vi "Receive Messages from Queue.vi"() -> ()   [LabVIEW 2015]
doc: "Demonstrates how to receive messages from an existing Amazon SQS queue."
uses:
  Core/HTTP Request/Region.ctl
  Core/HTTP Request/AWS Credentials.ctl
  Queue/Message.ctl
  Queue/Message Attribute Value Pair.ctl
  Queue/Message Attribute.ctl
  Queue/Custom Attribute.ctl
  Queue/Custom Attribute Type.ctl
  Queue/Queue Attribute.ctl
  Queue/Queue.lvclass
  Core/HTTP Request/HTTP Request.lvclass
panel:
  out "Messages":i32(listbox)
  in  "Region":T1
  in  "Secret Key":string
  in  "Access Key":string
  in  "Queue Name":string
  # "Overview: Demonstrates how to receive messages from an existing Amazon SQS queue.\nRequirements: LabVIEW AWS Toolkit and a registered Amazon AWS account\nInstructions:\n1. Specify the Access Key and Secret Key for your AWS account. You can create an account at http://aws.amazon.com.\n2. Specify a Region and Queue Name for the queue from which you want to receive messages.\n3. Run the VI. All the messages associated with your queue should be listed in the Messages indicator."
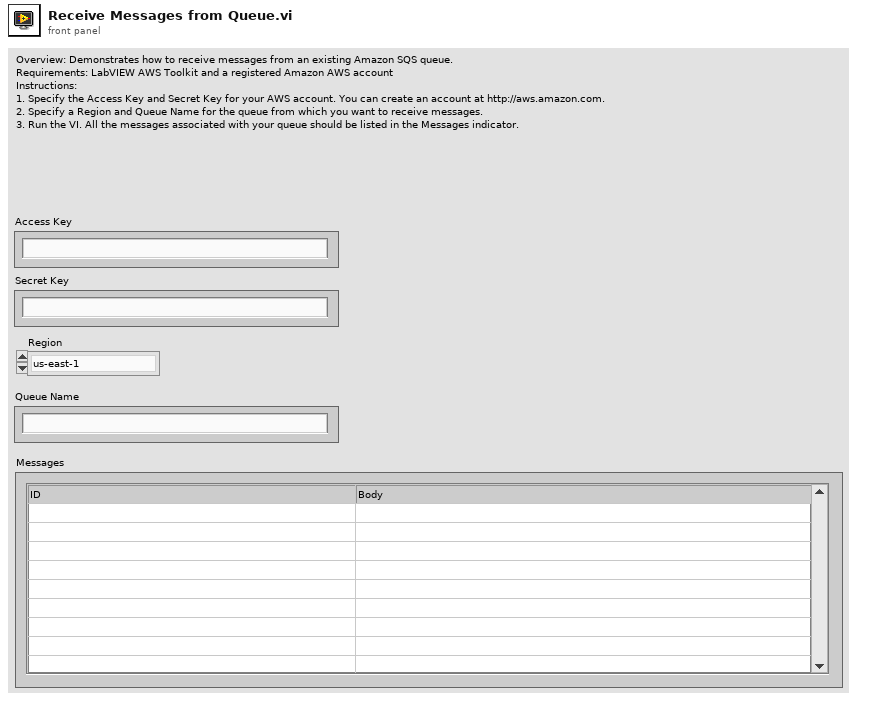
[diagram p1: front panel]
types:
  T1 = typedef "NI_AWS_Core.lvlib/HTTP Request.lvclass/Region.ctl" = enum16{"us-east-1", "us-east-2", "us-west-1", "us-west-2", "ap-northeast-1", "ap-northeast-2", "ap-southeast-1", "ap-southeast-2", "ca-central-1", "eu-central-1", "eu-west-1", "eu-west-2", "sa-east-1"}
  T2 = typedef "NI_AWS_SQS.lvlib/Queue.lvclass/Message.ctl" = cluster{"Body":string, "MD5 of Body":string, "ID":string, "Receipt Handle":string, "Native Attributes":T3[], "Custom Attributes":T5[], "MD5 of Custom Attributes":string}
  T3 = typedef "NI_AWS_SQS.lvlib/Queue.lvclass/Message Attribute Value Pair.ctl" = cluster{"Attribute":T4, "Value":string}
  T4 = typedef "NI_AWS_SQS.lvlib/Queue.lvclass/Message Attribute.ctl" = enum16{"SenderId", "SentTimestamp", "ApproximateReceiveCount", "ApproximateFirstReceiveTimestamp"}
  T5 = typedef "NI_AWS_SQS.lvlib/Queue.lvclass/Custom Attribute.ctl" = cluster{"Name":string, "Type":T6, "Value":string}
  T6 = typedef "NI_AWS_SQS.lvlib/Queue.lvclass/Custom Attribute Type.ctl" = enum16{"String", "Number", "Binary"}
  T7 = typedef "NI_AWS_Core.lvlib/HTTP Request.lvclass/AWS Credentials.ctl" = cluster{"Access Key":string, "Secret Key":string}
  T8 = typedef "NI_AWS_SQS.lvlib/Queue.lvclass/Queue Attribute Value Pair.ctl" = cluster{"Attribute":T9, "Value":string}
  T9 = typedef "NI_AWS_SQS.lvlib/Queue.lvclass/Queue Attribute.ctl" = enum16{"ApproximateNumberOfMessages", "ApproximateNumberOfMessagesDelayed", "ApproximateNumberOfMessagesNotVisible", "CreatedTimestamp", "DelaySeconds", "LastModifiedTimestamp", "MaximumMessageSize", "MessageRetentionPeriod", "Policy", "QueueArn", "ReceiveMessageWaitTimeSeconds", "RedrivePolicy", "VisibilityTimeout"}
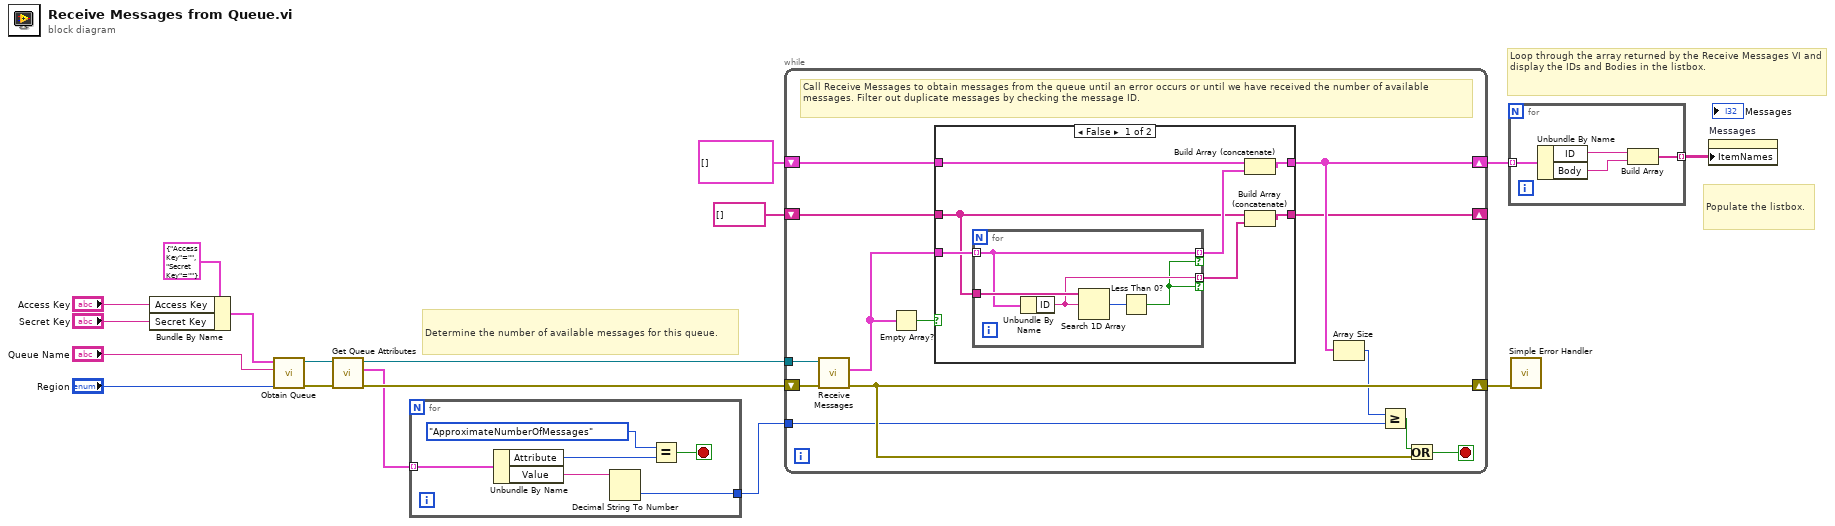
[diagram p0: block diagram]
diagram:
  # "Determine the number of available messages for this queue."
  # "Loop through the array returned by the Receive Messages VI and display the IDs and Bodies in the listbox."
  # "Populate the listbox."
  n1 = Bundle By Name(cluster=T7 {"Access Key"="", "Secret Key"=""} ("AWS Credentials"), "Access Key"="Access Key", "Secret Key"="Secret Key") -> (w14:T7)
  n2 = call "Obtain Queue.vi"("Region"="Region", "Name"="Queue Name", "AWS Credentials"=w14) -> ("error out"=w9:errorcluster, "SQS"=w7:refnum<class "Queue.lvclass">)  [unwired: 7 in]
  n3 = call "Get Queue Attributes.vi"("error in (no error)"=w9, "SQS in"=w7) -> ("error out"=w8:errorcluster, "Attribute Results"=w5:T8[], "SQS out"=w6:refnum<class "Queue.lvclass">)  [unwired: 7 in]
  n4 = for {
    tunnel: w5 -> [w23] mode=indexing
    tunnel: [w18] -> w2
    stop <- w20 stop-if-true
    n5 = Unbundle By Name(w23) -> ("Attribute"=w21:T9, "Value"=w19:string)
    n6 = Decimal String To Number(string=w19) -> (number=w18:i32)  [unwired: 2 in, 1 out]
    n7 = Equal?(x=Queue_Attribute."ApproximateNumberOfMessages" ("Attribute"), y=w21) -> (x = y?=w20:bool)
  }
  n8 = while {
    tunnel: w6 -> [w36]
    shift-right: [w34] -> w11
    shift-left: w8 -> [w35]
    shift-right: [w28] -> w3
    shift-left: T2[] [] ("Messages") -> [w32]
    tunnel: w2 -> [w29]
    shift-right: [w24] -> _
    shift-left: string[] [] ("Messages") -> [w25]
    stop <- w33 stop-if-true
    # "Call Receive Messages to obtain messages from the queue until an error occurs or until we have received the number of available messages. Filter out duplicate messages by checking the message ID."
    n9 = call "Receive Messages.vi"("error in (no error)"=w35, "SQS in"=w36) -> ("error out"=w34:errorcluster, "Messages"=w31:T2[])  [unwired: 7 in, 1 out]
    n10 = Empty Array?(array=w31) -> (empty?=w30:bool)
    n11 = case shown="False" w30 {
      tunnel: w32 -> [w43 w50]
      tunnel: w31 -> [w41 _]
      tunnel: [w42 w50] -> w28
      tunnel: w25 -> [w37 w49]
      tunnel: [w38 w49] -> w24
      frame False {
        n12 = for {
          tunnel: w41 -> [w46] mode=indexing
          tunnel: w37 -> [w48]
          tunnel: [w46] -> w40 mode=indexing if=w44
          tunnel: [w45] -> w39 mode=indexing if=w44
          n13 = Unbundle By Name(w46) -> ("ID"=w45:string)
          n14 = Search 1D Array(1D array=w48, element=w45) -> (index of element=w47:i32)  [unwired: 1 in]
          n15 = Less Than 0?(x=w47) -> (x < 0?=w44:bool)
        }
        n16 = Build Array (concatenate)(w43, w40) -> (w42:T2[])
        n17 = Build Array (concatenate)(w37, w39) -> (w38:string[])
      }
      frame True {
      }
    }
    n18 = Array Size(array=w28) -> (size(s)=w27:i32)
    n19 = Greater Or Equal?(x=w27, y=w29) -> (x >= y?=w26:bool)
    n20 = Or(x=w26, y=w34) -> (x .or. y?=w33:bool)
  }
  n21 = for {
    tunnel: w3 -> [w54] mode=indexing
    tunnel: [w51] -> w10 mode=indexing
    n22 = Unbundle By Name(w54) -> ("ID"=w53:string, "Body"=w52:string)
    n23 = Build Array(w53, w52) -> (w51:string[])
  }
  n24 = call <vilib>:"Simple Error Handler.vi"("error in (no error)"=w11) -> ()  [unwired: 4 in, 5 out]
  n25 = property on="Messages" class="MCListbox (strict)"("ItemNames"=w10) -> ()  [unwired: 2 in, 2 out]
